vi "Station Update For Duplicate IP.vi"(8 "error in (no error)":errorcluster, 11 "Connection Refnum":T1) -> (0 "error out":errorcluster, 2 "Stations with Dups":T2[](array[typedef]), 3 "Connection Refnum":T1)   [LabVIEW 2011]
uses:
  Station Record.ctl
  Summitek EXT/ODBC/SQL Controls/Connection Refnum.ctl
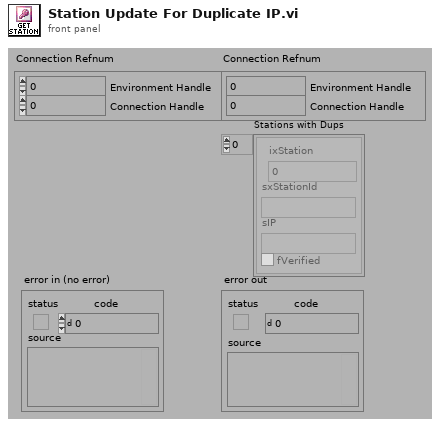
[diagram p1: front panel]
types:
  T1 = typedef "Connection Refnum.ctl" = cluster{"Environment Handle":i32, "Connection Handle":i32}
  T2 = typedef "Station Record.ctl" = cluster{"ixStation":i32, "sxStationId":string, "sIP":string, "fVerified":bool}
  T3 = typedef "Statement Refnum.ctl" = cluster{"Statement Handle":i32, "Parameter Number":u16}
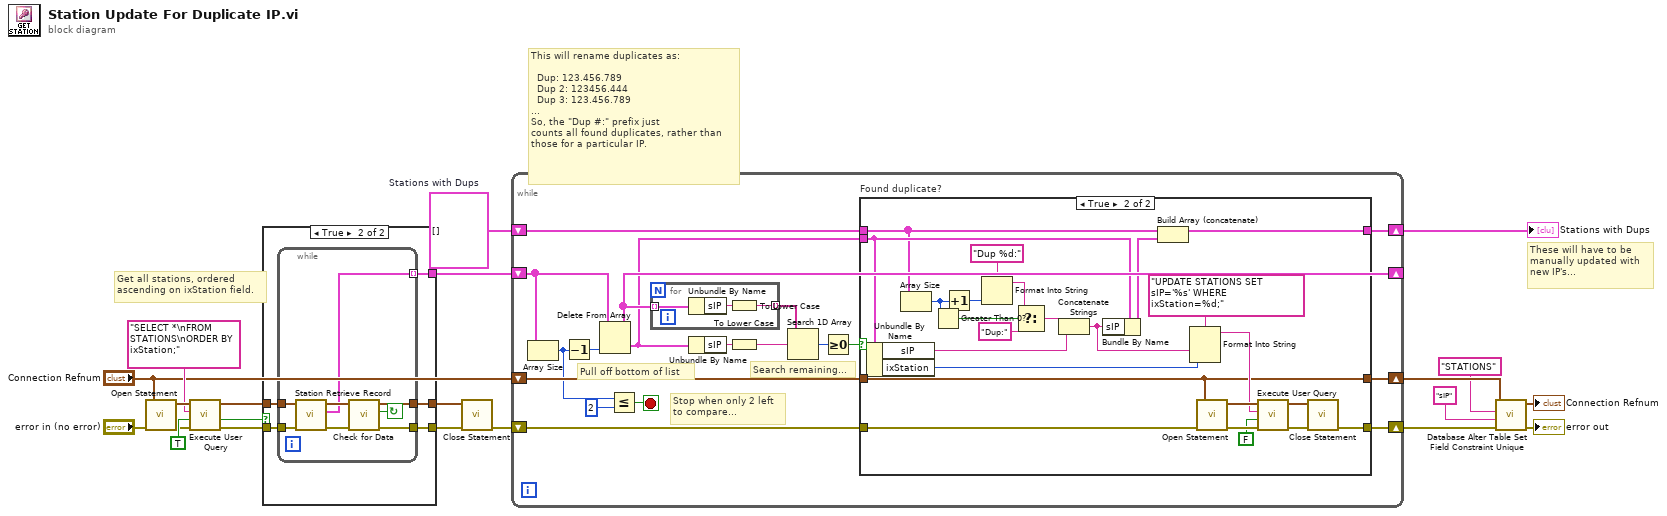
[diagram p0: block diagram]
diagram:
  w12 = T2[] []  # Stations with Dups
  # "This will rename duplicates as:\n\n  Dup: 123.456.789\n  Dup 2: 123456.444\n  Dup 3: 123.456.789\n...\nSo, the \"Dup #:\" prefix just\ncounts all found duplicates, rather than\nthose for a particular IP."
  # "These will have to be\nmanually updated with\nnew IP's..."
  # "Get all stations, ordered\nascending on ixStation field."
  n1 = call "Open Statement.vi"("error in (no error)"="error in (no error)", "Connection Refnum"="Connection Refnum") -> ("error out"=w16:errorcluster, "Statement Refnum"=w17:T3)  [unwired: 4 out]
  n2 = call "Execute User Query.vi"("error in (no error)"=w16, "Return Data? (f)"=TRUE, "User Query"="SELECT *\nFROM STATIONS\nORDER BY ixStation;" ("Query Name"), "Statement Refnum"=w17) -> ("error out"=w20:errorcluster, "Data Present?"=w21:bool, "Statement Refnum"=w19:T3)  [unwired: 1 out]
  n3 = case shown="True" w21 {
    tunnel: w20 -> [w22 w28]
    tunnel: w19 -> [w23 w27]
    tunnel: [w22 w26] -> w15
    tunnel: [w23 w25] -> w14
    tunnel: [_ w24] -> w9
    frame False {
    }
    frame True {
      n4 = while {
        tunnel: w28 -> [w30]
        tunnel: w27 -> [w33]
        tunnel: [w35] -> w26
        tunnel: [w34] -> w25
        tunnel: [w29] -> w24 mode=indexing
        stop <- w36 continue-if-true
        n5 = call "Station Retrieve Record.vi"("error in (no error)"=w30, "Statement Refnum"=w33) -> ("error out"=w31:errorcluster, "Station Record"=w29:T2, "Statement Refnum"=w32:T3)  [unwired: 7 out]
        n6 = call "Check for Data.vi"("error in (no error)"=w31, "Statement Refnum"=w32) -> ("error out"=w35:errorcluster, "Data Present?"=w36:bool, "Statement Refnum"=w34:T3)  [unwired: 3 out]
      }
    }
  }
  n7 = call "Close Statement.vi"("error in (no error)"=w15, "Statement Refnum"=w14) -> ("error out"=w10:errorcluster)  [unwired: 5 out]
  n8 = while {
    shift-right: [w51] -> w11
    shift-left: w12 -> [w52]
    shift-right: [w48] -> w8
    shift-left: "Connection Refnum" -> [w50]
    shift-right: [w47] -> w7
    shift-left: w10 -> [w49]
    shift-right: [w45] -> _
    shift-left: w9 -> [w46]
    stop <- w39 stop-if-true
    # "Search remaining..."
    # "Pull off bottom of list"
    # "Stop when only 2 left\nto compare..."
    n9 = Array Size(array=w46) -> (size(s)=w38:i32)
    n10 = Decrement(x=w38) -> (x-1=w40:i32)
    n11 = Delete From Array(array=w46, index=w40) -> (deleted portion=w41:T2, array with subset deleted=w45:T2[])  [unwired: 1 in]
    n12 = Less Or Equal?(x=w38, y=2) -> (x <= y?=w39:bool)
    n13 = for "For each station,\nfind matching IP's" {
      tunnel: w45 -> [w57] mode=indexing
      tunnel: [w55] -> w44 mode=indexing
      n14 = Unbundle By Name(w57) -> ("sIP"=w56:string)
      n15 = To Lower Case(string=w56) -> (all lower case string=w55:string)
    }
    n16 = Unbundle By Name(w41) -> ("sIP"=w43:string)
    n17 = To Lower Case(string=w43) -> (all lower case string=w42:string)
    n18 = Search 1D Array(1D array=w44, element=w42) -> (index of element=w54:i32)  [unwired: 1 out]
    n19 = Greater Or Equal To 0?(x=w54) -> (x >= 0?=w53:bool)
    n20 = case "Found duplicate?" shown="True" w53 {
      tunnel: w41 -> [_ w76]
      tunnel: w52 -> [w60 w64]
      tunnel: [w60 w84] -> w51
      tunnel: w50 -> [w58 w71]
      tunnel: w49 -> [w59 w78]
      tunnel: [w59 w77] -> w47
      tunnel: [w58 w71] -> w48
      frame False {
      }
      frame True {
        n21 = Unbundle By Name(w76) -> ("sIP"=w62:string, "ixStation"=w72:i32)
        n22 = Array Size(array=w64) -> (size(s)=w67:i32)
        n23 = Greater Than 0?(x=w67) -> (x > 0?=w66:bool)
        n24 = Increment(x=w67) -> (x+1=w65:i32)
        n25 = Format Into String(format string="Dup %d:", w65) -> (resulting string=w68:string)  [unwired: 2 in, 1 out]
        n26 = Select(t=w68, s=w66, f="Dup:") -> (s? t:f=w63:string)
        n27 = Concatenate Strings(w63, w62) -> (w61:string)
        n28 = Bundle By Name(cluster=w76, "sIP"=w61) -> (w75:T2)
        n29 = Build Array (concatenate)(w64, w75) -> (w84:T2[])
        n30 = Format Into String(format string="UPDATE STATIONS SET sIP='%s' WHERE ixStation=%d;" ("User Query"), w61, w72) -> (resulting string=w73:string)  [unwired: 2 in, 1 out]
        n31 = call "Open Statement.vi"("error in (no error)"=w78, "Connection Refnum"=w71) -> ("error out"=w82:errorcluster, "Statement Refnum"=w83:T3)  [unwired: 4 out]
        n32 = call "Execute User Query.vi"("error in (no error)"=w82, "Return Data? (f)"=FALSE, "User Query"=w73, "Statement Refnum"=w83) -> ("error out"=w80:errorcluster, "Statement Refnum"=w81:T3)  [unwired: 2 out]
        n33 = call "Close Statement.vi"("error in (no error)"=w80, "Statement Refnum"=w81) -> ("error out"=w77:errorcluster)  [unwired: 5 out]
      }
    }
  }
  "Stations with Dups" <- w11
  n34 = call "Database Alter Table Set Field Constraint Unique.vi"("error in (no error)"=w7, "Field (\"\")"="sIP" ("Table (\"\")"), "Table (\"\")"="STATIONS" ("Table (\"\")"), "Connection Refnum"=w8) -> ("error out"=→"error out":errorcluster, "Connection Refnum"=→"Connection Refnum":T1)  [unwired: 6 out]
